vi "PV ActiveLine - Gas Type Correction (TPG361).vi"(7 "W/R":bool, 8 "Fehler (Eingang)":errorcluster, 10 "Gas S 1":i8(ring) items=["Nitrogen", "Argon", "Hydrogen", "Helium", "Neon", "Krypton", "Xenon", "other"], 11 "Referenz in":refnum<visa-resource-name>) -> (0 "Cluster (Ausgang)":errorcluster, 2 "Gas Out 1":i8(ring) items=["Nitrogen", "Argon", "Hydrogen", "Helium", "Neon", "Krypton", "Xenon", "other"], 3 "Referenz out":refnum<visa-resource-name>)   [LabVIEW 2013, in "PV ActiveLine.lvlib"]
doc: "GAS – Gas Type Correction\n\nTransmit: GAS [a,a]\nReceive: a,a\n\nGas type correction,\na =\n0 –> nitrogen / air (default)\n1 –> Argon\n2 –> Hydrogen\n3 –> Helium\n4 –> Neon\n5 –> Krypton\n6 –> Xenon\n7 –> Other gases"
uses:
  <instrlib>/PV ActiveLine/PV ActiveLine.lvlib
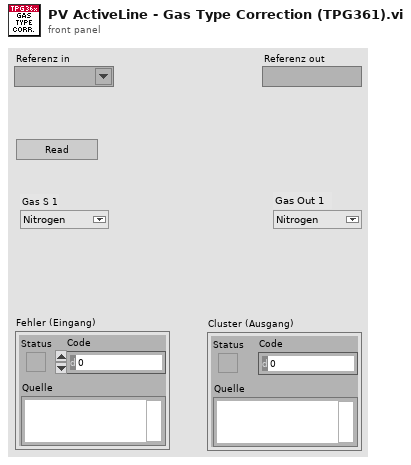
[diagram p1: front panel]
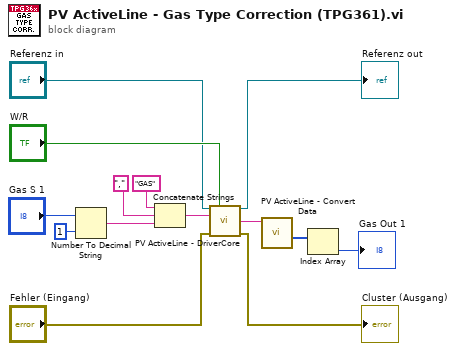
[diagram p0: block diagram]
diagram:
  n1 = Number To Decimal String(number="Gas S 1", width (-)=i16 1 ("Breite (-)")) -> (decimal integer string=w5:string)
  n2 = Concatenate Strings("GAS", "," ("String"), w5) -> (w8:string)
  n3 = call <instrlib>:"PV ActiveLine - DriverCore.vi"("Referenz in"="Referenz in", "Write/Read"="W/R", "Command"=w8, "Fehler (Eingang)"="Fehler (Eingang)") -> ("Referenz out"=→"Referenz out":refnum<visa-resource-name>, "String Out"=w3:string, "Cluster (Ausgang)"=→"Cluster (Ausgang)":errorcluster)  [unwired: 9 in]
  n4 = call <instrlib>:"PV ActiveLine - Convert Data.vi"("String in"=w3) -> ("Integer Out"=w2:i32[])  [unwired: 7 in, 3 out]
  n5 = Index Array(array=w2) -> (element=→"Gas Out 1":i32)  [unwired: 1 in]
